vi "PCA Read Data.vi"() -> (2 "Pitch":dbl, 3 "Roll":dbl)   [LabVIEW 2018]
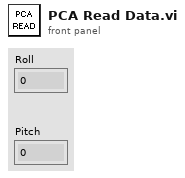
[diagram p1: front panel]
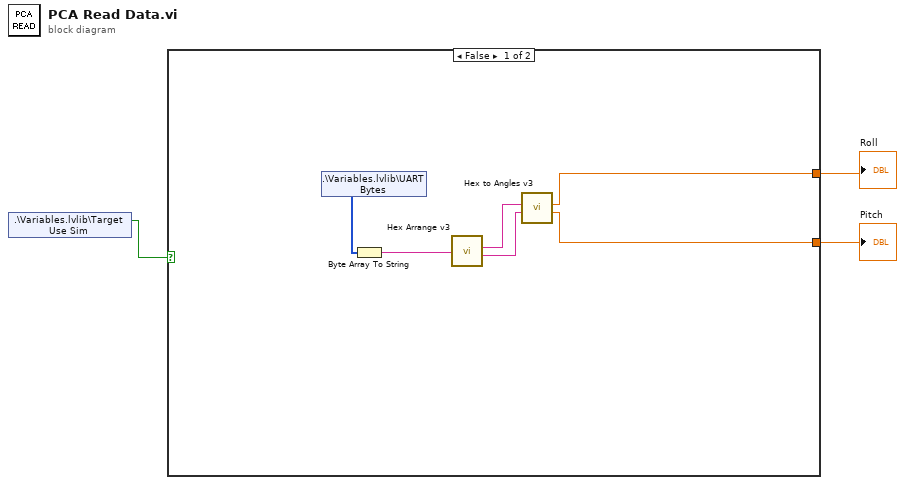
[diagram p0: block diagram]
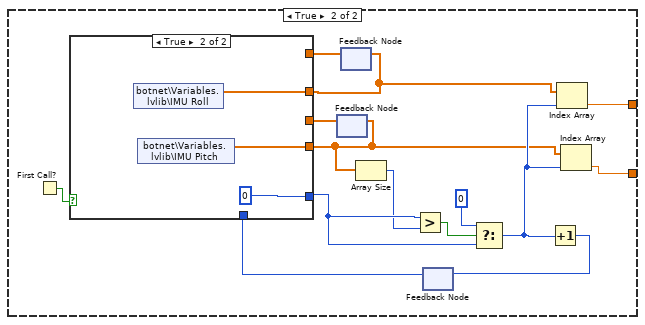
[diagram p2: hidden frame]
diagram:
  n1 = shared-variable ".\\Variables.lvlib\\Target Use Sim"() -> (w3:bool)  [unwired: 1 in, 1 out]
  n2 = case shown="False" w3 {
    tunnel: [w5 w11] -> w2
    tunnel: [w4 w10] -> w1
    frame False {
      n3 = shared-variable ".\\Variables.lvlib\\UART Bytes"() -> (w7:u8[])  [unwired: 1 in, 1 out]
      n4 = Byte Array To String(unsigned byte array=w7) -> (string=w6:string)
      n5 = call "Hex Arrange v3.vi"("Hex from UART"=w6) -> ("after substring"=w9:string, "Corrected Hex"=w8:string)  [unwired: 9 in]
      n6 = call "Hex to Angles v3.vi"("Hex after Headers"=w9, "Hex from UART"=w8) -> ("Pitch Angle [rad]"=w4:dbl, "Roll Angle [rad]"=w5:dbl)  [unwired: 7 in, 1 out]
    }
    frame True {
      n7 = First Call?() -> (First Call?: T/F=w13:bool)
      n8 = feedback #1() -> (w22:dbl[])  [unwired: 1 in]
      n9 = feedback #2() -> (w23:dbl[])  [unwired: 1 in]
      n10 = feedback #3() -> (w20:i32)  [unwired: 1 in]
      n11 = case shown="True" w13 {
        tunnel: [w26 w29] -> w15
        tunnel: w23 -> [w26 _]
        tunnel: [w25 w28] -> w12
        tunnel: w22 -> [w25 _]
        tunnel: [w24 0] -> w17
        tunnel: w20 -> [w24 _]
        frame False {
        }
        frame True {
          n12 = shared-variable "botnet\\Variables.lvlib\\IMU Roll"() -> (w29:dbl[])  [unwired: 1 in, 1 out]
          n13 = shared-variable "botnet\\Variables.lvlib\\IMU Pitch"() -> (w28:dbl[])  [unwired: 1 in, 1 out]
        }
      }
      n14 = feedback-in #1(w12) -> ()
      n15 = feedback-in #2(w15) -> ()
      n16 = Array Size(array=w12) -> (size(s)=w16:i32)
      n17 = Greater?(x=w17, y=w16) -> (0:w18:bool)
      n18 = Select(t=0, s=w18, f=w17) -> (s? t:f=w14:i32)
      n19 = Increment(x=w14) -> (x+1=w21:i32)
      n20 = feedback-in #3(w21) -> ()
      n21 = Index Array(array=w15, index=w14) -> (element=w11:dbl)
      n22 = Index Array(array=w12, index=w14) -> (element=w10:dbl)
    }
  }
  "Roll" <- w2
  "Pitch" <- w1
